vi "Wrapper_getSpectrum_Mod.vi"(8 "error in (no error)":errorcluster caption="entrée d'erreur (pas d'erreur)", 10 "Wrapper":u32, 11 "Index":i32) -> (0 "error out":errorcluster caption="sortie d'erreur", 1 "Length":i32, 2 "Spectrum Values":dbl[](array[numeric]))   [LabVIEW 2024]
uses:
  common32.dll
  OmniDriver32.dll
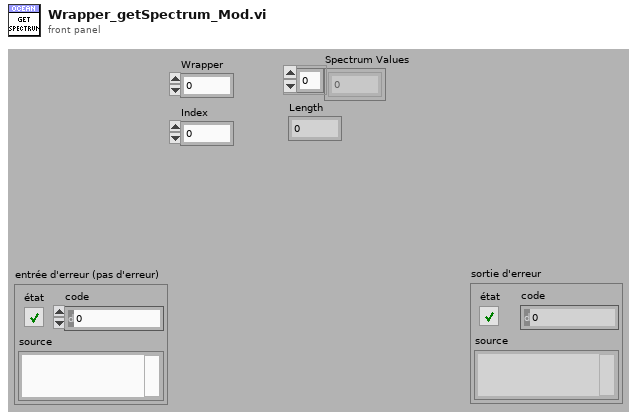
[diagram p1: front panel]
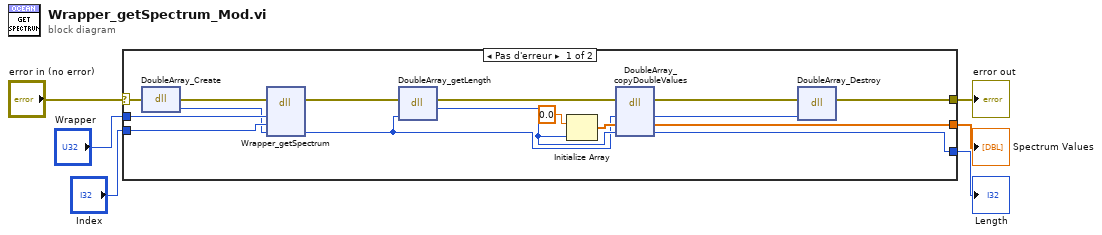
[diagram p0: block diagram]
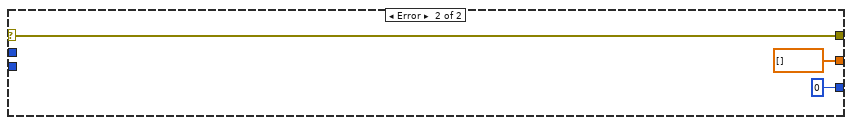
[diagram p2: hidden frame]
diagram:
  n1 = case shown="Pas d'erreur" "error in (no error)" {
    selector: "error in (no error)" -> [w12 w23]
    tunnel: "Wrapper" -> [w22 _]
    tunnel: "Index" -> [w21 _]
    tunnel: [w15 dbl[] [] ("Values")] -> w4
    tunnel: [w14 0 ("Length")] -> w3
    tunnel: [w7 w23] -> w1
    frame No Error {
      n2 = dll-call lib="common32.dll" fn="DoubleArray_Create" label="DoubleArray.Create"(error in=w12) -> (error out=w11:errorcluster, "return type"=w20:u32)  [unwired: 2 in, 1 out]
      n3 = dll-call lib="OmniDriver32.dll" fn="Wrapper_getSpectrum" label="Wrapper.getSpectrum"(error in=w11, "Wrapper"=w22, "Index"=w21, "DoubbleArray"=w20) -> (error out=w10:errorcluster, "DoubbleArray"=w16:u32)  [unwired: 4 in, 2 out]
      n4 = dll-call lib="common32.dll" fn="DoubleArray_getLength" label="DoubleArray.getLength"(error in=w10, "DoubbleArray"=w16) -> (error out=w9:errorcluster, "return type"=w17:i32)  [unwired: 3 in, 1 out]
      n5 = Initialize Array(0.0 ("element"), w17) -> (w18:dbl[])
      n6 = dll-call lib="common32.dll" fn="DoubleArray_copyDoubleValues" label="DoubleArray.copyDoubleValues"(error in=w9, "DoubbleArray"=w16, "Values"=w18, "Length"=w17) -> (error out=w8:errorcluster, "DoubbleArray"=w13:u32, "Values"=w15:dbl[], "Length"=w14:i32)  [unwired: 2 in, 2 out]
      n7 = dll-call lib="common32.dll" fn="DoubleArray_Destroy" label="DoubleArray.Destroy"(error in=w8, "DoubleArray"=w13) -> (error out=w7:errorcluster)  [unwired: 3 in, 2 out]
    }
    frame Error {
    }
  }
  "Spectrum Values" <- w4
  "Length" <- w3
  "error out" <- w1
